vi "King Swap 3.vi"(0 "1D Board":T2[](array[typedef]), 5 "DT Team #":i32, 11 "error in (no error)":errorcluster) -> (4 "1D Board Out":T2[](array[typedef]), 6 "Cell to move to":i32, 8 "Output Text":string, 15 "error out":errorcluster)   [LabVIEW 2014]
uses:
  Typedefs/Board Cell.ctl
  Typedefs/Cell Occupancy.ctl
  Typedefs/Select Empty DT or Both.ctl
  Dragon Tamers.lvlib
panel:
  in  "Enum":T1=enum."Empty and DT"
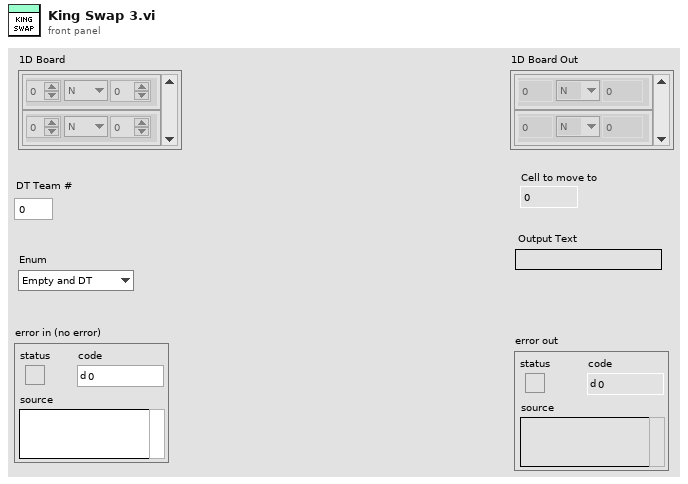
[diagram p1: front panel]
types:
  T1 = typedef "Select Empty DT or Both.ctl" = enum16{"Empty Only", "DT Cells Only", "Empty and DT"}
  T2 = typedef "Dragon Tamers.lvlib/Board Cell.ctl" = cluster{"Team":i32, "Occu.":T3, "Count":i32}
  T3 = typedef "Dragon Tamers.lvlib/Cell Occupancy.ctl" = enum16{"N", "C", "K"}
  T4 = typedef "Dragon Tamers.lvlib/Parsed Board.ctl" = cluster{"DT King":i32, "Opp King":i32, "Count":i32[], "Empty Cells":i32[], "DT Cells":i32[], "Opp Cells":i32[], "DT Team":i32, "Opp. Team":i32}
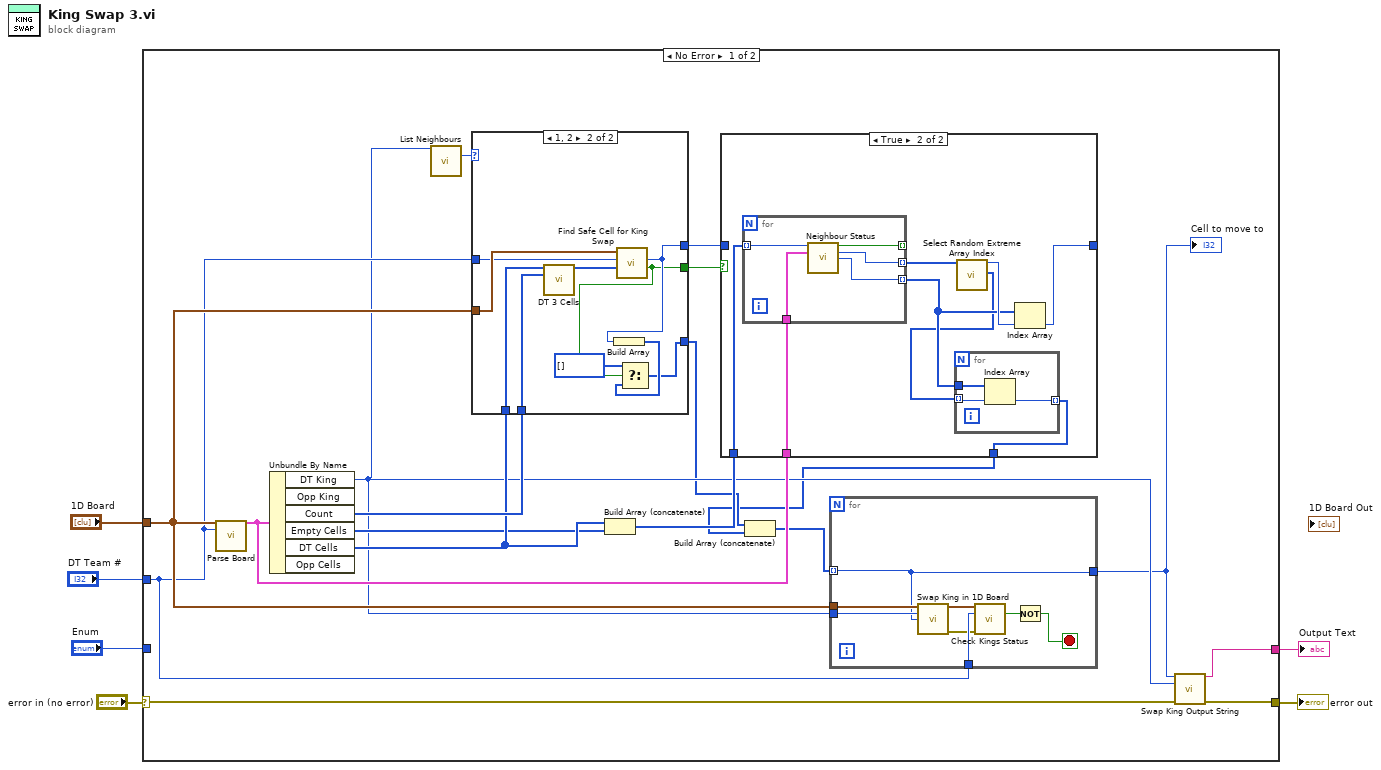
[diagram p0: block diagram]
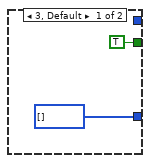
[diagram p3: hidden frame]
diagram:
  n1 = case shown="No Error" "error in (no error)" {
    selector: "error in (no error)" -> [w23 w62]
    tunnel: [w24 w62] -> w5
    tunnel: "1D Board" -> [w13 _]
    tunnel: "DT Team #" -> [w12 _]
    tunnel: [w22 _] -> w2
    tunnel: "Enum" -> [_ _]
    frame No Error {
      n2 = call "Parse Board.vi"("Board Array"=w13, "DT Team #"=w12) -> ("Parsed Board Info"=w18:T4)  [unwired: 12 in, 1 out]
      n3 = Unbundle By Name(w18) -> ("DT King"=w11:i32, "Count"=w21:i32[], "Empty Cells"=w15:i32[], "DT Cells"=w16:i32[])  [unwired: 2 out]
      n4 = call "List Neighbours.vi"("Cell Index"=w11) -> ("Max Capacity"=w20:i32)  [unwired: 12 in, 2 out]
      n5 = case shown="1, 2" w20 {
        tunnel: w16 -> [_ w61]
        tunnel: w21 -> [_ w60]
        tunnel: w13 -> [_ w59]
        tunnel: w12 -> [_ w57]
        tunnel: [TRUE ("Empty Array?") w55] -> w19
        tunnel: [_ w56] -> w17
        tunnel: [i32[] [] w52] -> w10
        frame 3, Default {
        }
        frame 1, 2 {
          n6 = call "DT 3 Cells.vi"("DT 3 Cells"=w61, "Count"=w60) -> ("DT 3 Cells"=w58:i32[])  [unwired: 11 in, 2 out]
          n7 = call "Find Safe Cell for King Swap.vi"("Candidate Cells"=w58, "DT Team #"=w57, "1D Board"=w59) -> ("Empty Array?"=w55:bool, "Selected Cell"=w56:i32)  [unwired: 6 in, 1 out]
          n8 = Build Array(w56) -> (w54:i32[])
          n9 = Select(t=i32[] [], s=w55, f=w54) -> (s? t:f=w52:i32[])
        }
      }
      n10 = Build Array (concatenate)(w16, w15) -> (w14:i32[])
      n11 = case shown="True" w19 {
        tunnel: w18 -> [_ w38]
        tunnel: w17 -> [w33 _]
        tunnel: [w33 w39] -> _
        tunnel: w14 -> [_ w37]
        tunnel: [_ w34] -> w9
        frame False {
        }
        frame True {
          n12 = for {
            tunnel: w38 -> [w49]
            tunnel: [w48] -> _ mode=indexing
            tunnel: [w47] -> w40 mode=indexing
            tunnel: [w46] -> w36 mode=indexing
            tunnel: w37 -> [w45] mode=indexing
            n13 = call "Neighbour Status.vi"("Cell"=w45, "Parsed Board"=w49) -> ("Full?"=w48:bool, "Min Count to Max"=w47:i32, "Cell Index"=w46:i32)  [unwired: 10 in, 1 out]
          }
          n14 = call "Select Random Extreme Array Index.vi"("Array"=w40) -> ("Chosen Max Index"=w41:i32, "Max[]"=w35:i32[])  [unwired: 14 in, 3 out]
          n15 = for {
            tunnel: w36 -> [w44]
            tunnel: w35 -> [w43] mode=indexing
            tunnel: [w42] -> w34 mode=indexing
            n16 = Index Array(array=w44, index=w43) -> (element=w42:i32)
          }
          n17 = Index Array(array=w36, index=w41) -> (element=w39:i32)
        }
      }
      n18 = Build Array (concatenate)(w10, w9) -> (w8:i32[])
      n19 = for {
        tunnel: w13 -> [w32]
        tunnel: w12 -> [w30]
        tunnel: w11 -> [w28]
        tunnel: w8 -> [w25] mode=indexing
        tunnel: [w25] -> w7
        stop <- w26 stop-if-true
        n20 = call "Swap King in 1D Board.vi"("1D Board"=w32, "King Index"=w28, "Cell Index"=w25) -> ("1D Board Out"=w31:T2[], "error out"=w29:errorcluster)  [unwired: 11 in]
        n21 = call "Check Kings Status.vi"("1D Board"=w31, "DT Team"=w30, "error in (no error)"=w29) -> ("DT King in Danger?"=w27:bool)  [unwired: 7 in, 5 out]
        n22 = Not(x=w27) -> (.not. x?=w26:bool)
      }
      "Cell to move to" <- w7
      n23 = call "Swap King Output String.vi"("New Cell Index"=w7, "Old Cell Index"=w11, "error in (no error)"=w23) -> ("Output Text"=w22:string, "error out"=w24:errorcluster)  [unwired: 11 in]
    }
    frame Error {
    }
  }
  "error out" <- w5
  "Output Text" <- w2
